vi "Init.vi"(8 "error in (no error)":errorcluster, 10 "Last Update (None)":timestamp, 11 "Path":path) -> (0 "error out":errorcluster, 3 "ViaApp out":refnum<class "ViaApp.lvclass">)   [LabVIEW 2020, in "PicoG-App.lvlib" / "ViaApp.lvclass"]
uses:
  ViaApp.lvclass
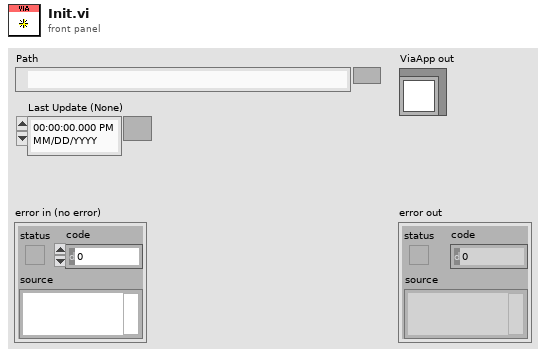
[diagram p1: front panel]
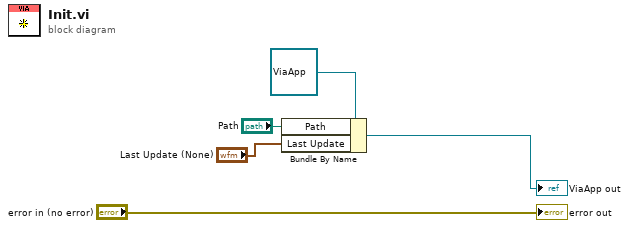
[diagram p0: block diagram]
diagram:
  n1 = Bundle By Name(cluster=refnum<class "ViaApp.lvclass"> refnum ("ViaApp in"), "Path"="Path", "Last Update"="Last Update (None)") -> (→"ViaApp out":refnum<class "ViaApp.lvclass">)
  "error out" <- "error in (no error)"
